vi "Chroma 1905x Series Source Settings in Step.vi"(8 "error in (no error)":errorcluster, 11 "VISA resource name":refnum<visa-resource-name>) -> (0 "error out":errorcluster, 2 "Settings":string, 3 "VISA resource name out":refnum<visa-resource-name>)   [LabVIEW 2025]
doc: "Chroma\n5 Clock Tower Place Suite 210\nMaynard, MA 01754\nTel: 1 800 253-1230\nTel: 1 877 4 A HIPOT\nFax: 1 978-461-4295\nWebsite: www.chroma.com"
panel:
  in  "Step":u32=1 min=1 max=99 step=1
  # "Settings by Step"
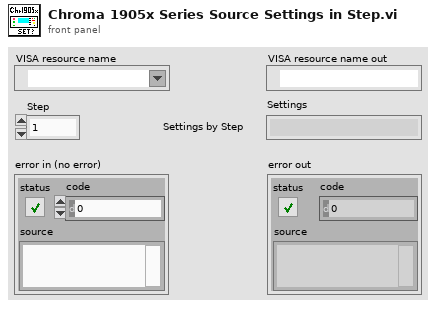
[diagram p1: front panel]
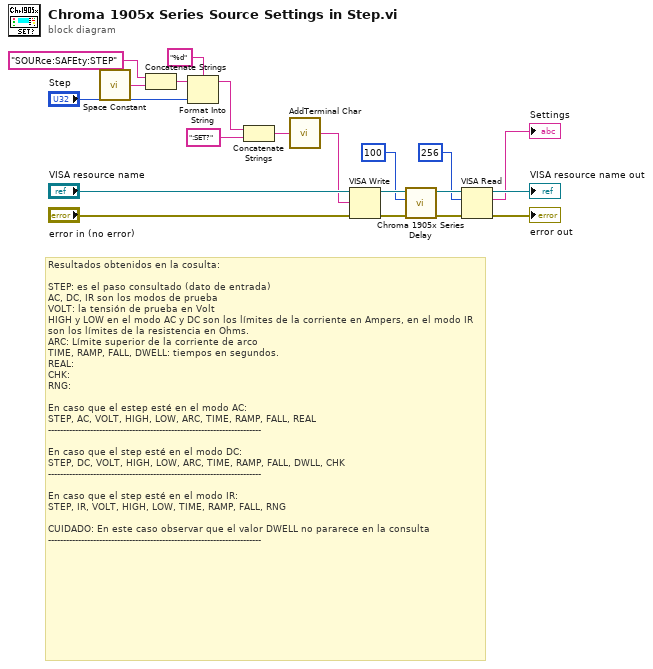
[diagram p0: block diagram]
diagram:
  # "Resultados obtenidos en la cosulta:\n\nSTEP: es el paso consultado (dato de entrada)\nAC, DC, IR son los modos de prueba\nVOLT: la tensión de prueba en Volt\nHIGH y LOW en el modo AC y DC son los límites de la corriente en Ampers, en el modo IR son los límites de la resistencia en Ohms.\nARC: Límite superior de la corriente de arco\nTIME, RAMP, FALL, DWELL: tiempos en segundos.\nREAL: \nCHK:\nRNG:\n\nEn caso que el estep esté en el modo AC:\nSTEP, AC, VOLT, HIGH, LOW, ARC, TIME, RAMP, FALL, REAL\n-----------------------------------------------------------------------\n\nEn caso que el step esté en el modo DC:\nSTEP, DC, VOLT, HIGH, LOW, ARC, TIME, RAMP, FALL, DWLL, CHK\n-----------------------------------------------------------------------\n\nEn caso que el step esté en el modo IR:\nSTEP, IR, VOLT, HIGH, LOW, TIME, RAMP, FALL, RNG\n\nCUIDADO: En este caso observar que el valor DWELL no pararece en la consulta\n-----------------------------------------------------------------------"
  n1 = call <vilib>:"Space Constant.vi"() -> ("String"=w2:string)
  n2 = Concatenate Strings("SOURce:SAFEty:STEP", w2) -> (w1:string)
  n3 = Format Into String(format string="%d", initial string=w1, "Step") -> (resulting string=w6:string)  [unwired: 1 in, 1 out]
  n4 = Concatenate Strings(w6, ":SET?") -> (w4:string)
  n5 = call "AddTerminal Char.vi"("Cmd string"=w4) -> ("Concatenated String"=w12:string)  [unwired: 4 in]
  n6 = VISA Write(VISA resource name="VISA resource name", write buffer=w12, error in (no error)="error in (no error)") -> (VISA resource name out=w18:refnum<visa-resource-name>, error out=w20:errorcluster)  [unwired: 1 out]
  n7 = call "Chroma 1905x Series Delay.vi"("error in (no error)"=w20, "Time Delay [ms]"=u32 100 ("Time Delay ms"), "VISA resource name"=w18) -> ("error out"=w19:errorcluster, "VISA resource name 2"=w17:refnum<visa-resource-name>)  [unwired: 7 in]
  n8 = VISA Read(VISA resource name=w17, byte count=u32 256, error in (no error)=w19) -> (VISA resource name out=→"VISA resource name out":refnum<visa-resource-name>, read buffer=→"Settings":string, error out=→"error out":errorcluster)  [unwired: 1 out]
